vi "Index Array (Boolean Value).vi"(8 "error in (no error)":errorcluster, 9 "index":i32, 10 "JSON Array in":refnum<class "JSON Helper.lvclass">) -> (0 "error out":errorcluster, 1 "Boolean":bool)   [LabVIEW 2016, in "JSON Helper.lvclass"]
doc: "Returns the Boolean value of the JSON Boolean element of the JSON array at index."
uses:
  JSON Helper/JSON Helper.lvclass
  Index Array (JSON).vi
  JSON Boolean/Read value (Boolean).vi
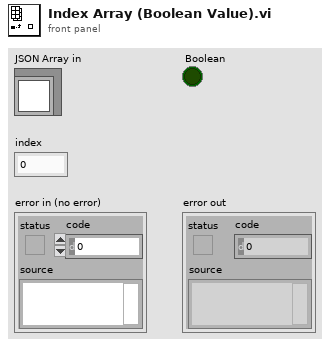
[diagram p1: front panel]
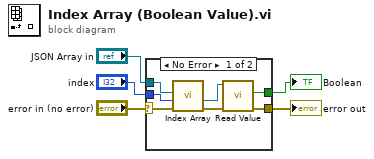
[diagram p0: block diagram]
diagram:
  n1 = case shown="No Error" "error in (no error)" {
    selector: "error in (no error)" -> [w8 w13]
    tunnel: [w9 w13] -> w4
    tunnel: "JSON Array in" -> [w7 _]
    tunnel: "index" -> [w6 _]
    tunnel: [w10 _] -> w1
    frame No Error {
      n2 = call-poly "Index Array.vi"("error in"=w8, "index"=w6, "JSON Array in"=w7) -> ("error out"=w11:errorcluster, "JSON out"=w12:refnum<class "JSON Helper.lvclass">)  [unwired: 7 in]
      n3 = call-poly "Read Value.vi"("error in (no error)"=w11, "JSON Boolean in"=w12) -> ("error out"=w9:errorcluster, "value"=w10:bool)  [unwired: 8 in]
    }
    frame Error {
    }
  }
  "error out" <- w4
  "Boolean" <- w1
